vi "Path Type -- Enum.vi"(1 "Value":path) -> (0 "Enum":T1(ring))   [LabVIEW 2017]
doc: "Classifies a path as an absolute path, a relative path or <Not A Path>."
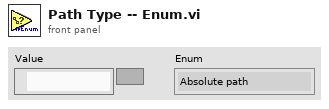
[diagram p1: front panel]
types:
  T1 = enum16{"Absolute path", "Relative path", "<Not A Path>"}
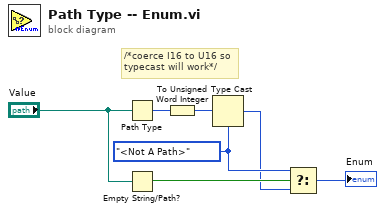
[diagram p0: block diagram]
diagram:
  w4 = T1."<Not A Path>"
  # "/*coerce I16 to U16 so typecast will work*/"
  n1 = Path Type(1:"Value") -> (0:w7:i16)
  n2 = Empty String/Path?(string/path="Value") -> (empty?=w5:bool)
  n3 = To Unsigned Word Integer(number=w7) -> (unsigned 16bit integer=w1:u16)
  n4 = Type Cast(type=w4, x=w1) -> (*(type *) &x=w3:T1)
  n5 = Select(t=w4, s=w5, f=w3) -> (s? t:f=→"Enum":T1)
